vi "VendingMachine.vi"() -> ()   [LabVIEW 2019]
uses:
  Control_typedef.ctl
  Enum_states.ctl
panel:
  out "Progress":u8(slide) scale=0.0..100.0
  in  "?":bool
  in  "?":bool
  in  "?":bool
  in  "?":bool
  in  "?":bool
  in  "?":bool
  in  "Wallet":T1
  out "Juice":dbl(slide) scale=0.0..2000.0
  out "Water":dbl(slide) scale=0.0..2000.0
  out "Rum":dbl(slide) scale=0.0..2000.0
  out "Lime":dbl(slide) scale=0.0..2000.0
  out "Sugar":dbl(slide) scale=0.0..2000.0
  out "Coke":dbl(slide) scale=0.0..2000.0
  out "Whisky":dbl(slide) scale=0.0..2000.0
  in  "?":bool
  in  "?":bool
  in  "Maintainance":bool
  out "string cluster":T2
  out "Boolean":bool
  in  "ON/OFF":bool
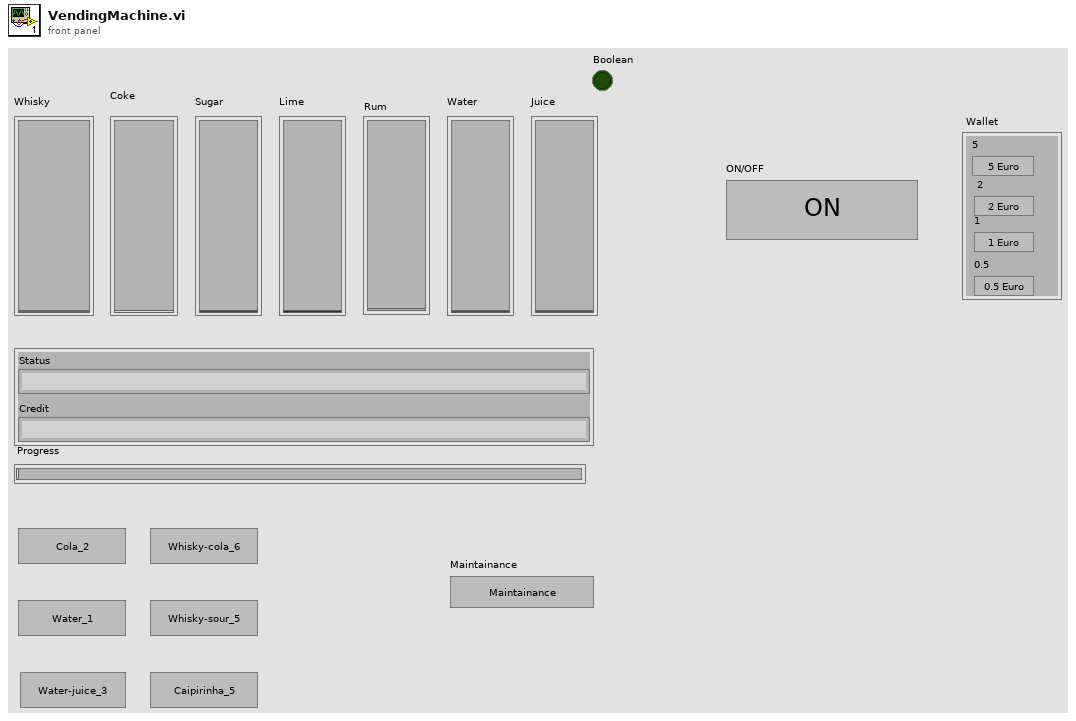
[diagram p1: front panel]
types:
  T1 = cluster{"5":bool, " 2":bool, "1":bool, "0.5":bool}
  T2 = typedef "Control_typedef.ctl" = cluster{"Status":string, "Credit":string}
  T3 = typedef "Enum_states.ctl" = enum16{"Cola-WaitMessage", "caipirinha", "whisky-sour", "whisky-cola", "water-juice", "water", "cola", "add0.5", "add1", "add2", "add5", "initialize", "OFF", "Admin mode", "Refill", "stop"}
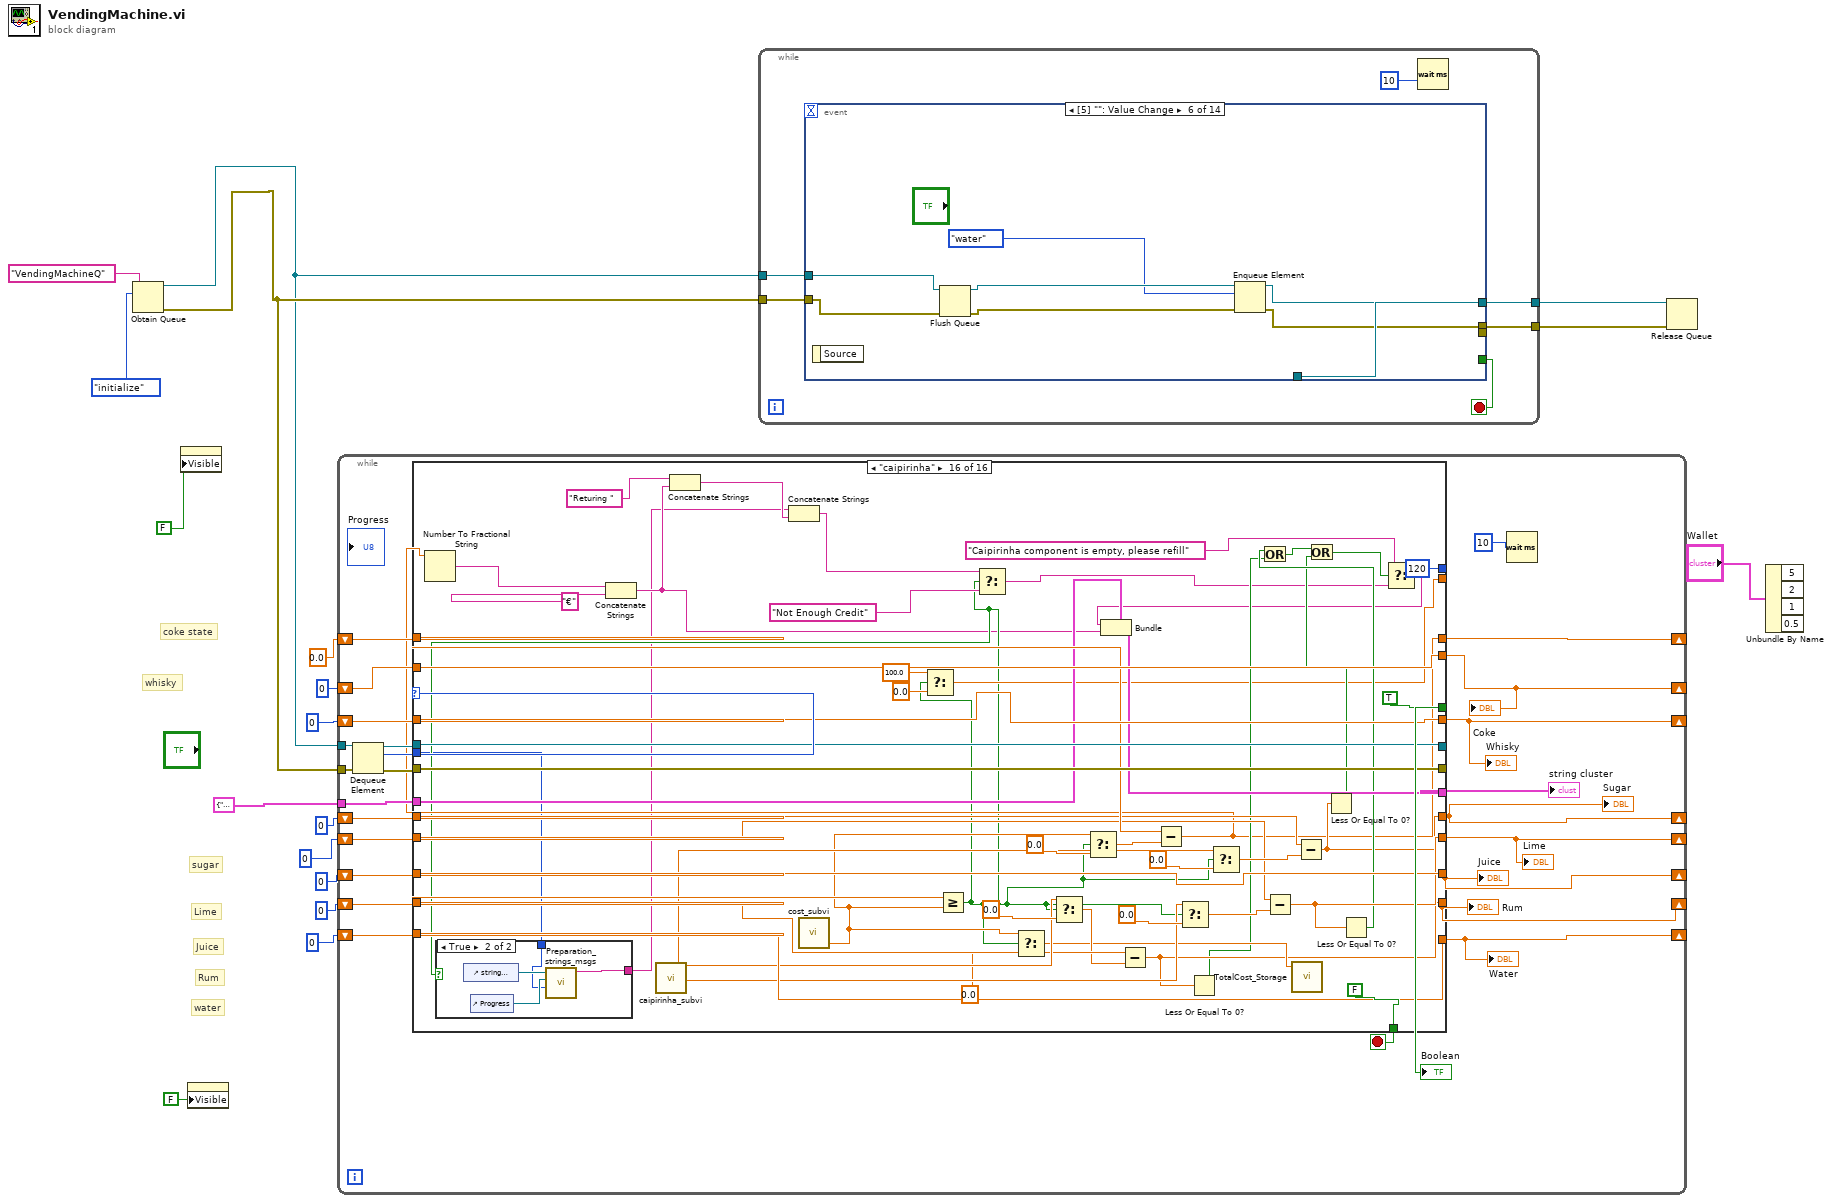
[diagram p0: block diagram]
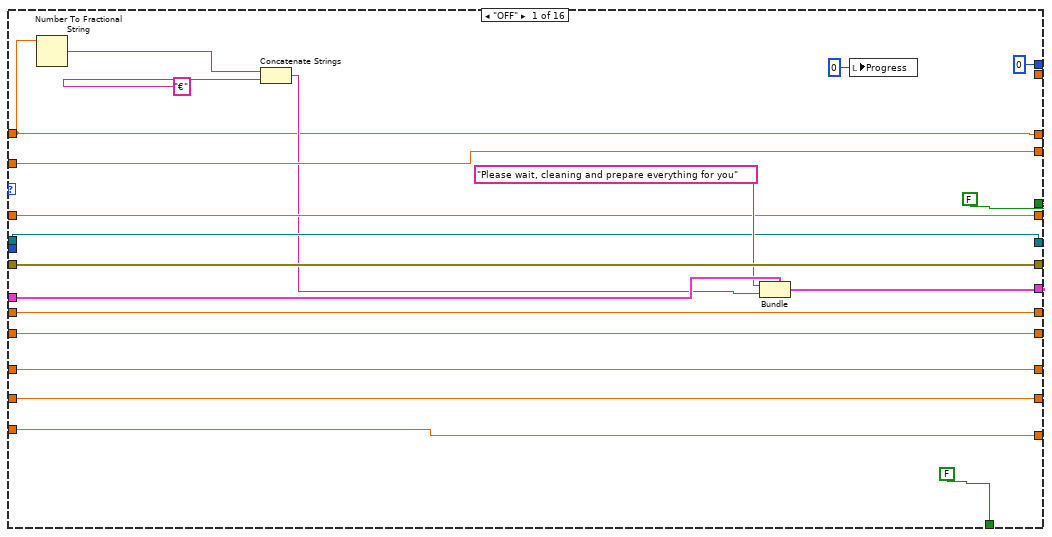
[diagram p2: hidden frame]
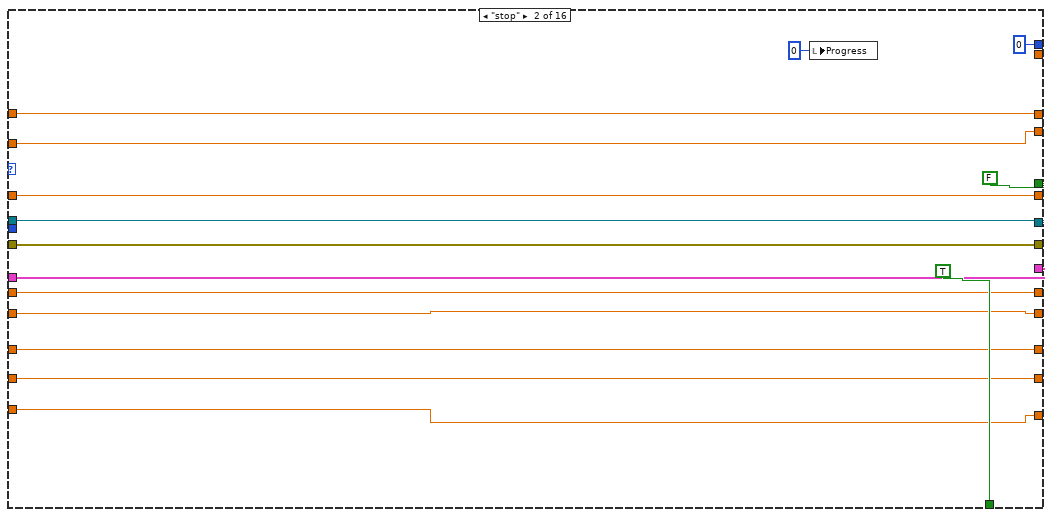
[diagram p3: hidden frame]
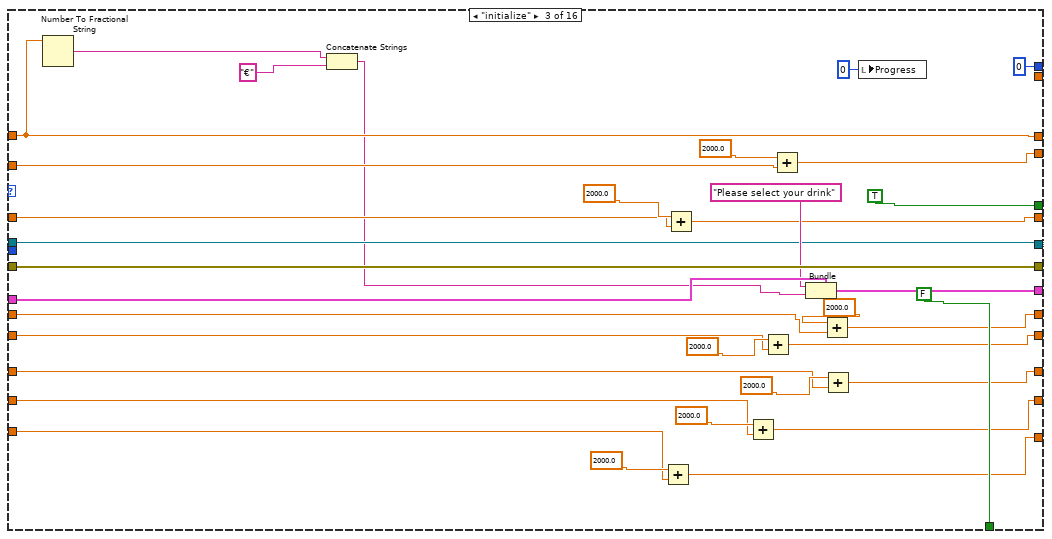
[diagram p4: hidden frame]
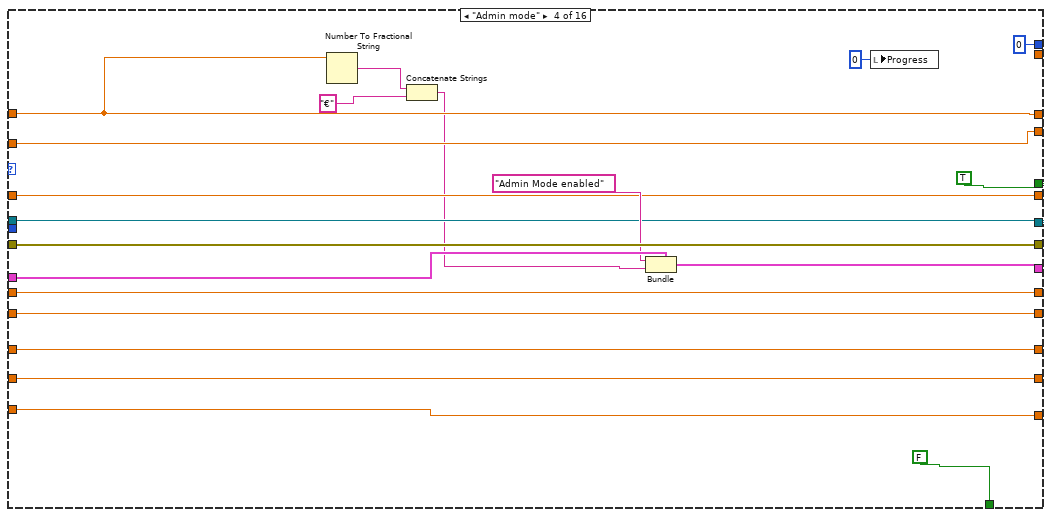
[diagram p5: hidden frame]
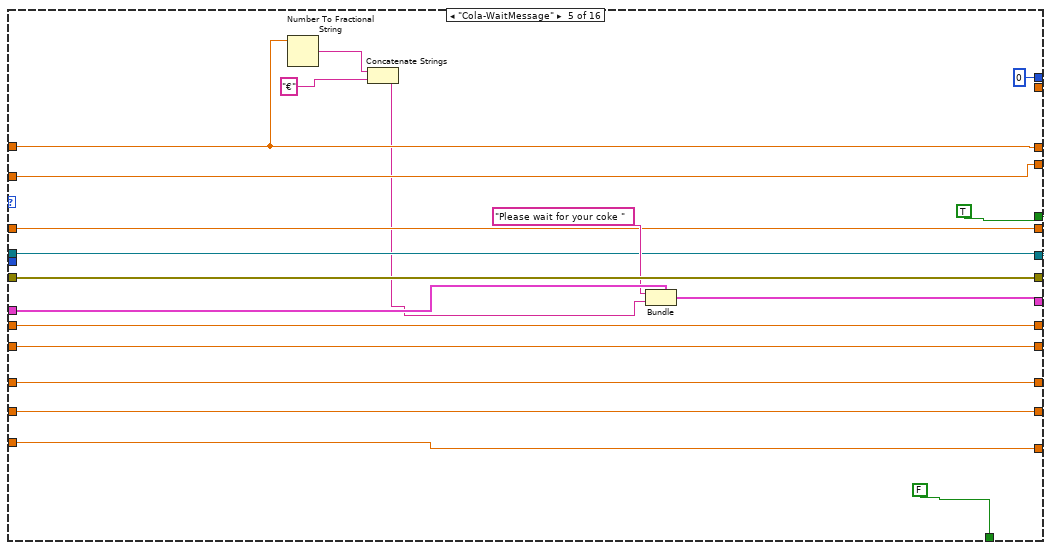
[diagram p6: hidden frame]
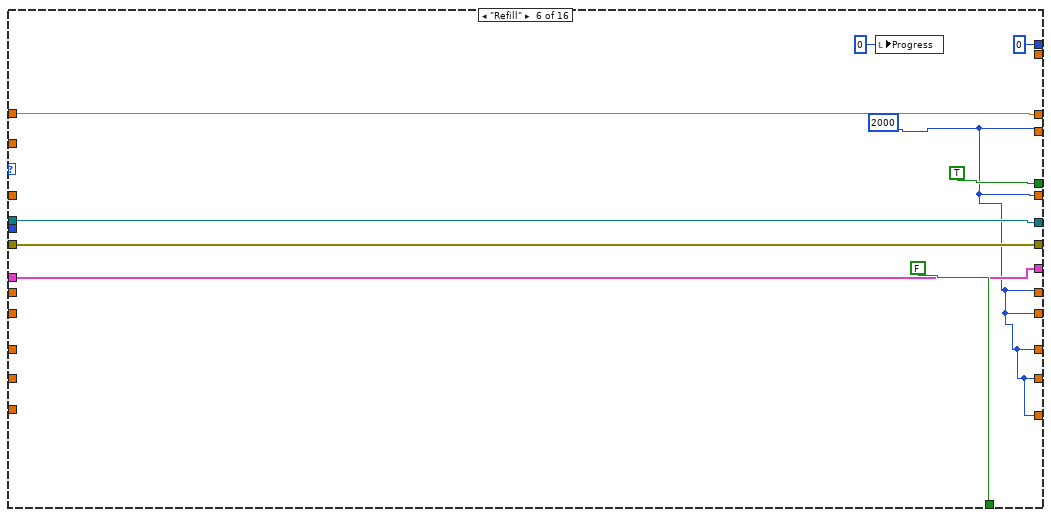
[diagram p7: hidden frame]
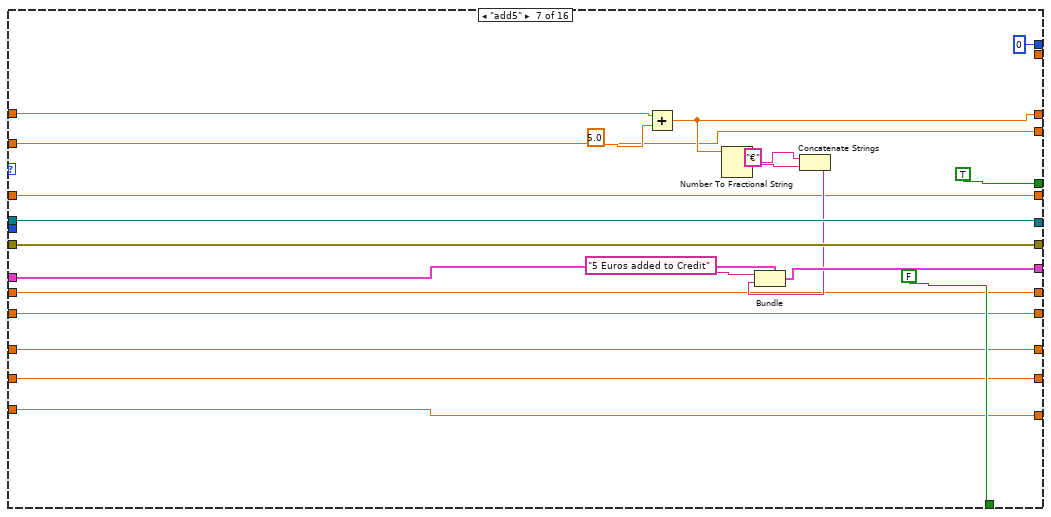
[diagram p8: hidden frame]
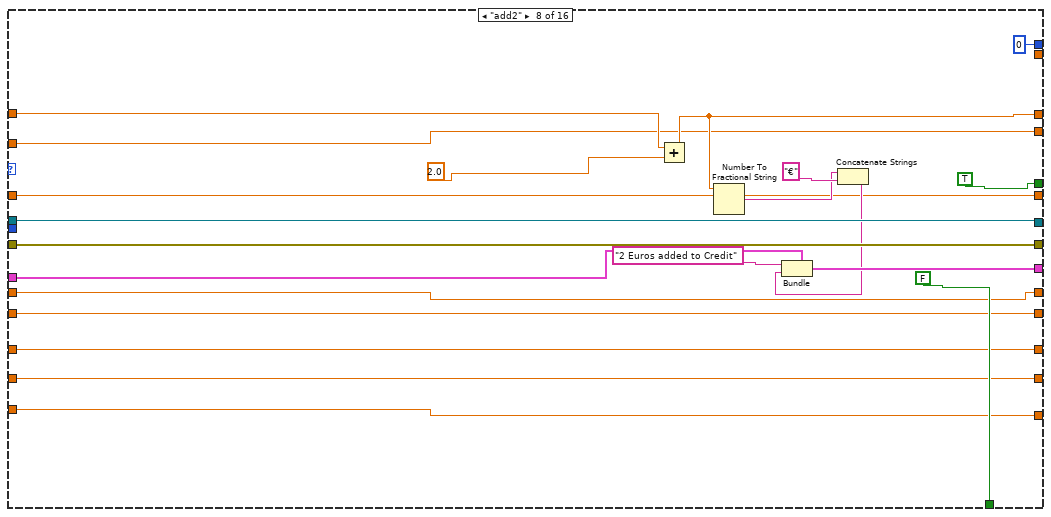
[diagram p9: hidden frame]
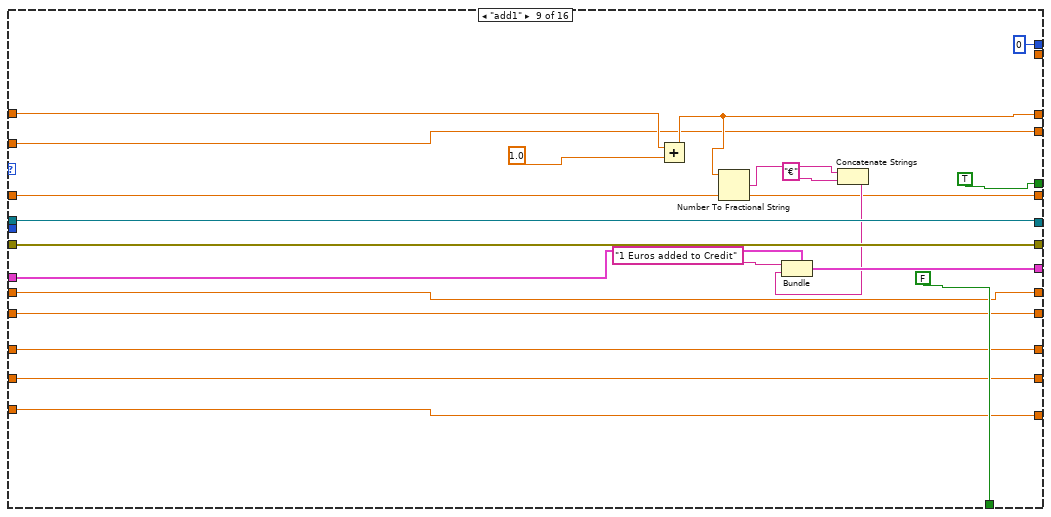
[diagram p10: hidden frame]
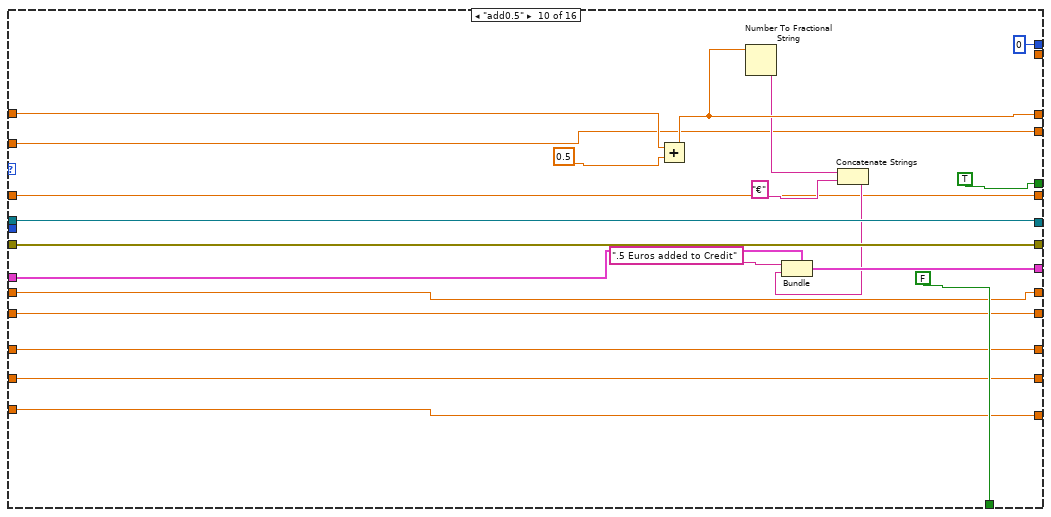
[diagram p11: hidden frame]
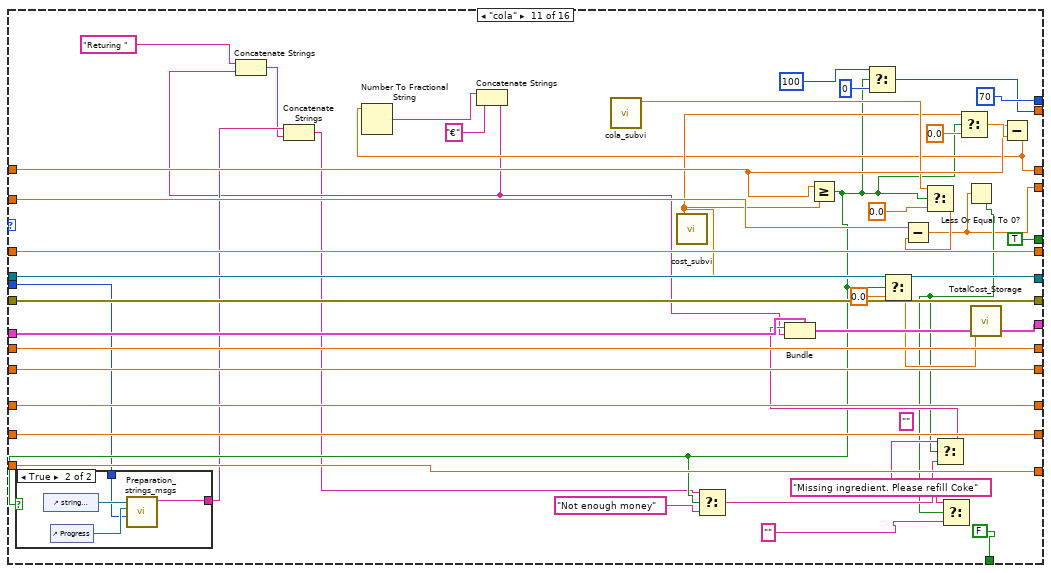
[diagram p12: hidden frame]
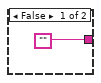
[diagram p13: hidden frame]
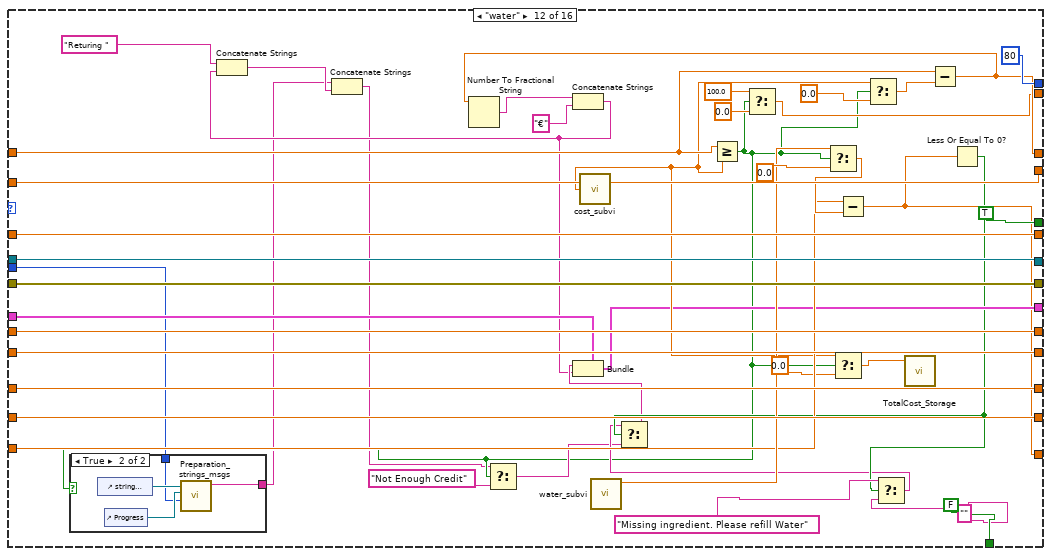
[diagram p14: hidden frame]
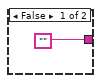
[diagram p15: hidden frame]
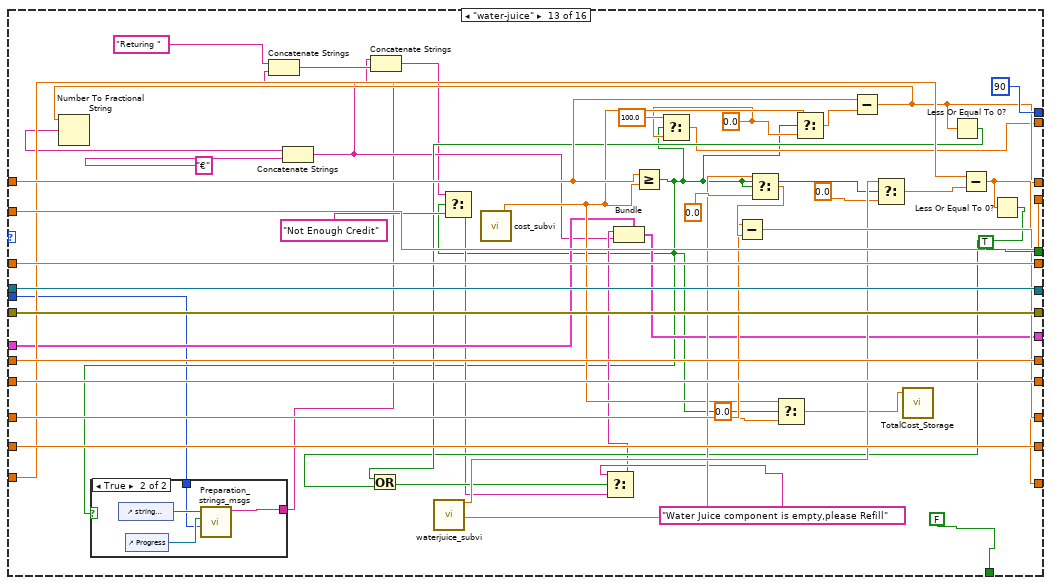
[diagram p16: hidden frame]
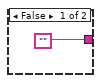
[diagram p17: hidden frame]
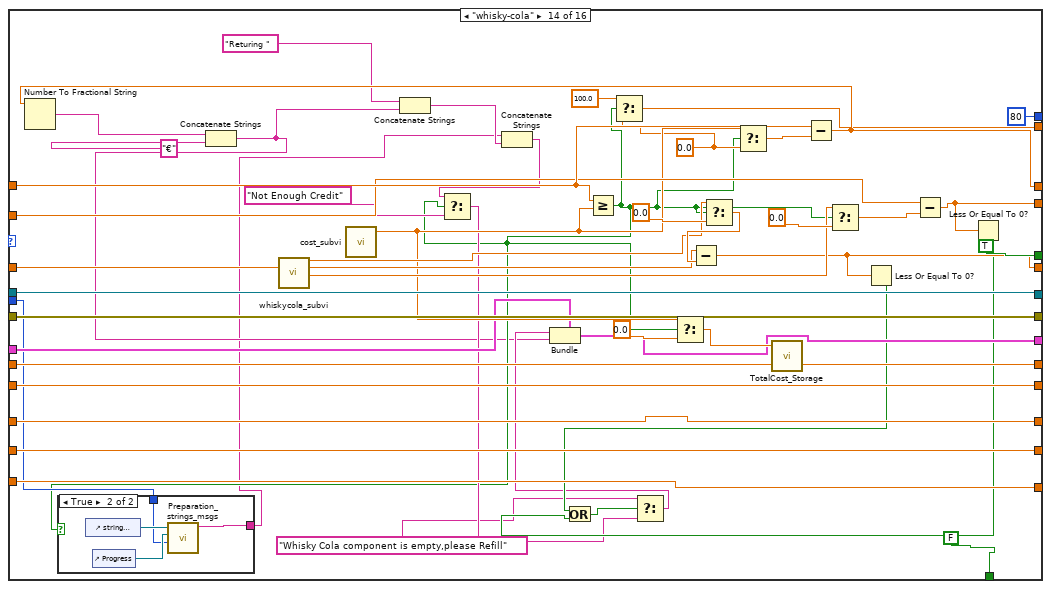
[diagram p18: hidden frame]
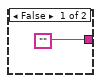
[diagram p19: hidden frame]
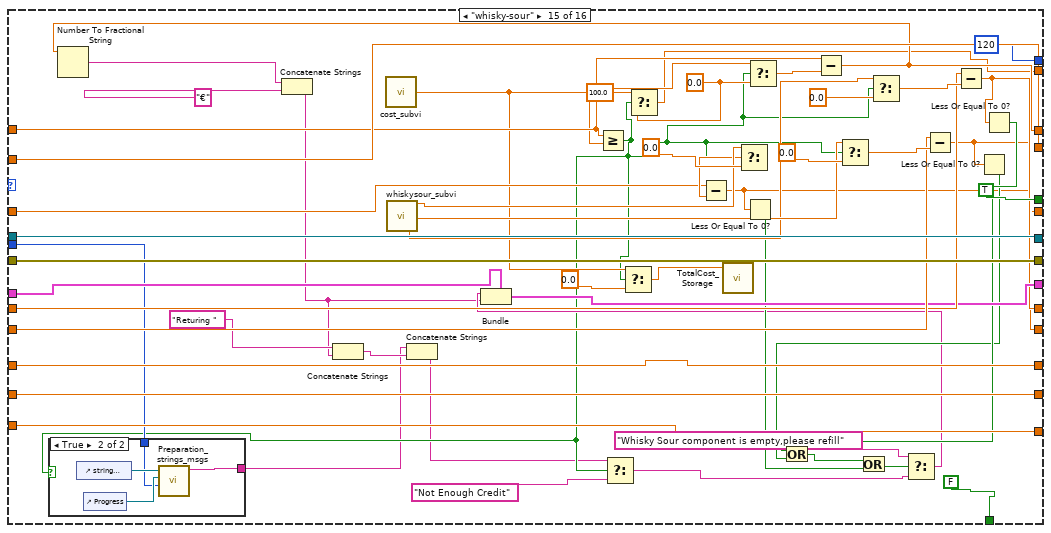
[diagram p20: hidden frame]
diagram:
  # "whisky"
  # "water"
  # "Rum"
  # "Juice"
  # "Lime"
  # "sugar"
  # "coke state"
  n1 = Obtain Queue(name (unnamed)="VendingMachineQ", element data type=Enum_states."initialize") -> (queue out=w12:refnum<queue>, error out=w13:errorcluster)  [unwired: 3 in, 1 out]
  n2 = property class="Bool"("Visible"=FALSE) -> ()  [unwired: 2 in, 2 out]
  n3 = property class="Bool"("Visible"=FALSE) -> ()  [unwired: 2 in, 2 out]
  n4 = while {
    tunnel: w12 -> [w44]
    tunnel: w13 -> [w43]
    tunnel: cluster{string, string} {"", ""} -> [w39]
    shift-right: [w35] -> _
    shift-left: 0.0 -> [w34]
    shift-right: [w32] -> _
    shift-left: 0 -> [w33]
    shift-right: [w26] -> _
    shift-left: 0 -> [w31]
    shift-right: [w27] -> _
    shift-left: 0 -> [w30]
    shift-right: [w28] -> _
    shift-left: 0 -> [w29]
    shift-right: [w24] -> _
    shift-left: 0 -> [w25]
    shift-right: [w22] -> _
    shift-left: 0 -> [w23]
    shift-right: [w20] -> _
    shift-left: 0 -> [w21]
    stop <- w37 stop-if-true
    n5 = Dequeue Element(queue=w44, error in (no error)=w43) -> (queue out=w41:refnum<queue>, element=w36:T3, error out=w40:errorcluster)  [unwired: 1 in, 1 out]
    n6 = case shown="\"caipirinha\"" w36 {
      tunnel: [FALSE FALSE TRUE TRUE TRUE TRUE TRUE TRUE TRUE TRUE TRUE TRUE TRUE TRUE TRUE TRUE] -> w42
      tunnel: w41 -> [w59 w75 w108 w128 w147 w160 w182 w203 w224 w245 w288 w337 w389 w433 w493 w554]
      tunnel: w40 -> [w64 w76 w112 w133 w152 w161 w181 w202 w223 w244 w287 w336 w388 w441 w499 w558]
      tunnel: [w64 w76 w112 w133 w152 w161 w181 w202 w223 w244 w287 w336 w388 w441 w499 w558] -> _
      tunnel: w39 -> [w63 w77 w111 w130 w149 w157 w176 w197 w218 w239 w271 w317 w365 w418 w474 w531]
      tunnel: [w62 w77 w109 w131 w150 w157 w175 w196 w217 w238 w270 w316 w364 w417 w473 w530] -> w38
      tunnel: [FALSE TRUE FALSE FALSE FALSE FALSE FALSE FALSE FALSE FALSE FALSE FALSE FALSE FALSE FALSE FALSE] -> w37
      tunnel: [w59 w75 w108 w128 w147 w160 w182 w203 w224 w245 w288 w337 w389 w433 w493 w554] -> _
      tunnel: [w54 w70 w104 w123 w142 w155 w166 w190 w208 w232 w260 w325 w383 w414 w492 w553] -> w32
      tunnel: w36 -> [_ _ _ _ _ _ _ _ _ _ w252 w300 w348 w401 w453 w510]
      tunnel: w34 -> [w46 w74 w82 w116 w135 w156 w177 w199 w220 w241 w273 w323 w377 w427 w487 w544]
      tunnel: [w46 w74 w82 w116 w135 w156 w171 w192 w213 w234 w258 w306 w353 w406 w458 w516] -> w35
      tunnel: w33 -> [w54 w70 w105 w123 w142 _ w166 w190 w208 w232 w284 w325 w383 w423 w492 w553]
      tunnel: w31 -> [w57 w73 w90 w126 w145 _ w169 w189 w211 w231 w283 w333 w385 w438 w478 w537]
      tunnel: w30 -> [w56 w72 w96 w125 w144 _ w168 w188 w210 w230 w282 w332 w376 w434 w494 w539]
      tunnel: [w55 w71 w98 w124 w143 w155 w167 w187 w209 w229 w281 w331 w384 w437 w496 w527] -> w28
      tunnel: w29 -> [w55 w71 w99 w124 w143 _ w167 w187 w209 w229 w281 w331 w384 w437 w496 w542]
      tunnel: [w56 w72 w95 w125 w144 w155 w168 w188 w210 w230 w282 w332 w375 w434 w494 w539] -> w27
      tunnel: [w57 w73 w89 w126 w145 w155 w169 w189 w211 w231 w283 w333 w385 w438 w471 w524] -> w26
      tunnel: w25 -> [w53 w69 w87 w122 w141 _ w165 w186 w207 w228 w280 w330 w382 w425 w484 w552]
      tunnel: [w53 w69 w86 w122 w141 w155 w165 w186 w207 w228 w280 w330 w382 w416 w466 w552] -> w24
      tunnel: w23 -> [w52 w68 w102 w121 w140 _ w164 w185 w206 w227 w279 w321 w370 w435 w495 w555]
      tunnel: [w52 w68 w101 w121 w140 w155 w164 w185 w206 w227 w279 w314 w363 w435 w495 w555] -> w22
      tunnel: w21 -> [w51 w67 w93 w120 w139 _ w163 w184 w205 w226 w278 w329 w381 w436 w482 w536]
      tunnel: [w51 w67 w92 w120 w139 w155 w163 w184 w205 w226 w278 w329 w381 w436 w469 w529] -> w20
      tunnel: [u32 0 ("milliseconds to wait") u32 0 ("milliseconds to wait") u32 0 ("milliseconds to wait") u32 0 ("milliseconds to wait") u32 0 ("milliseconds to wait") u32 0 ("milliseconds to wait") u32 0 ("milliseconds to wait") u32 0 ("milliseconds to wait") u32 0 ("milliseconds to wait") u32 0 ("milliseconds to wait") u32 70 ("milliseconds to wait") u32 80 ("milliseconds to wait") u32 90 ("milliseconds to wait") u32 80 ("milliseconds to wait") u32 120 ("milliseconds to wait") u32 120 ("milliseconds to wait")] -> _
      tunnel: [_ _ _ _ _ _ _ _ _ _ w255 w303 w350 w402 w454 w512] -> _
      frame "OFF" {
        n7 = Number To Fractional String(number=w46) -> (F-format string=w48:string)  [unwired: 3 in]
        n8 = Concatenate Strings(w48, "€" ("string")) -> (w47:string)
        n9 = Bundle(cluster=w63, "Please wait, cleaning and prepare everything for you", w47) -> (w62:cluster{string, string})
        n10 = local write "Progress"(u8 0 ("Progress")) -> ()
      }
      frame "stop" {
        n11 = local write "Progress"(u8 0 ("Progress")) -> ()
      }
      frame "initialize" {
        n12 = Number To Fractional String(number=w82) -> (F-format string=w83:string)  [unwired: 3 in]
        n13 = Concatenate Strings(w83, "€" ("string")) -> (w81:string)
        n14 = Add(x=2000.0, y=w102) -> (x+y=w101:dbl)
        n15 = Add(x=2000.0, y=w87) -> (x+y=w86:dbl)
        n16 = Add(x=2000.0, y=w99) -> (x+y=w98:dbl)
        n17 = Add(x=2000.0, y=w93) -> (x+y=w92:dbl)
        n18 = Add(x=2000.0, y=w105) -> (x+y=w104:dbl)
        n19 = Bundle(cluster=w111, "Please select your drink", w81) -> (w109:cluster{string, string})
        n20 = Add(x=2000.0, y=w90) -> (x+y=w89:dbl)
        n21 = Add(x=2000.0, y=w96) -> (x+y=w95:dbl)
        n22 = local write "Progress"(u8 0 ("Progress")) -> ()
      }
      frame "Admin mode" {
        n23 = Number To Fractional String(number=w116) -> (F-format string=w117:string)  [unwired: 3 in]
        n24 = Concatenate Strings(w117, "€" ("string")) -> (w115:string)
        n25 = Bundle(cluster=w130, "Admin Mode enabled", w115) -> (w131:cluster{string, string})
        n26 = local write "Progress"(u8 0 ("Progress")) -> ()
      }
      frame "Cola-WaitMessage" {
        n27 = Number To Fractional String(number=w135) -> (F-format string=w136:string)  [unwired: 3 in]
        n28 = Concatenate Strings(w136, "€" ("string")) -> (w134:string)
        n29 = Bundle(cluster=w149, "Please wait for your coke ", w134) -> (w150:cluster{string, string})
      }
      frame "Refill" {
        w155 = 2000
        n30 = local write "Progress"(u8 0 ("Progress")) -> ()
      }
      frame "add5" {
        n31 = Add(x=w177, y=5.0) -> (x+y=w171:dbl)
        n32 = Number To Fractional String(number=w171) -> (F-format string=w170:string)  [unwired: 3 in]
        n33 = Concatenate Strings(w170, "€" ("string")) -> (w172:string)
        n34 = Bundle(cluster=w176, "5 Euros added to Credit", w172) -> (w175:cluster{string, string})
      }
      frame "add2" {
        n35 = Add(x=w199, y=2.0) -> (x+y=w192:dbl)
        n36 = Number To Fractional String(number=w192) -> (F-format string=w191:string)  [unwired: 3 in]
        n37 = Concatenate Strings(w191, "€" ("string")) -> (w195:string)
        n38 = Bundle(cluster=w197, "2 Euros added to Credit", w195) -> (w196:cluster{string, string})
      }
      frame "add1" {
        n39 = Add(x=w220, y=1.0) -> (x+y=w213:dbl)
        n40 = Number To Fractional String(number=w213) -> (F-format string=w212:string)  [unwired: 3 in]
        n41 = Concatenate Strings(w212, "€" ("string")) -> (w216:string)
        n42 = Bundle(cluster=w218, "1 Euros added to Credit", w216) -> (w217:cluster{string, string})
      }
      frame "add0.5" {
        n43 = Add(x=w241, y=0.5) -> (x+y=w234:dbl)
        n44 = Number To Fractional String(number=w234) -> (F-format string=w233:string)  [unwired: 3 in]
        n45 = Concatenate Strings(w233, "€" ("string")) -> (w237:string)
        n46 = Bundle(cluster=w239, ".5 Euros added to Credit", w237) -> (w238:cluster{string, string})
      }
      frame "cola" {
        (unwired) ""
        w263 = "Missing ingredient. Please refill Coke"
        n47 = call "cola_subvi.vi"() -> ("volume"=w272:dbl)  [unwired: 9 in, 2 out]
        n48 = call "cost_subvi.vi"() -> ("Cola"=w268:dbl)  [unwired: 5 out]
        n49 = Greater Or Equal?(x=w273, y=w268) -> (x >= y?=w253:bool)
        n50 = case shown="True" w253 {
          tunnel: ["" w292] -> w251
          tunnel: w252 -> [_ w290]
          frame False {
          }
          frame True {
            n51 = control-ref of="string cluster"() -> (w293:refnum<vi>)
            n52 = control-ref of="Progress"() -> (w291:refnum<vi>)
            n53 = call "Preparation_strings_msgs.vi"("Enum"=w290, "reference"=w291, "Cluster in"=w293) -> ("Status"=w292:string)  [unwired: 8 in]
          }
        }
        n54 = Select(t=100, s=w253, f=0) -> (s? t:f=w255:i32)
        n55 = Select(t=w268, s=w253, f=0.0) -> (s? t:f=w266:dbl)
        n56 = Select(t=w272, s=w253, f=0.0) -> (s? t:f=w276:dbl)
        n57 = Subtract(x=w284, y=w276) -> (x-y=w260:dbl)
        n58 = Select(t=w268, s=w253, f=0.0) -> (s? t:f=w274:dbl)
        n59 = Less Or Equal To 0?(x=w260) -> (x <= 0?=w261:bool)
        n60 = Select(t=w263, s=w261, f="") -> ()  [unwired: 1 out]
        n61 = call "TotalCost_Storage.vi"("Numeric"=w266) -> ()  [unwired: 11 in]
        n62 = Subtract(x=w273, y=w274) -> (x-y=w258:dbl)
        n63 = Number To Fractional String(number=w258) -> (F-format string=w257:string)  [unwired: 3 in]
        n64 = Concatenate Strings(w257, "€" ("string")) -> (w249:string)
        n65 = Concatenate Strings("Returing " ("string"), w249) -> (w247:string)
        n66 = Concatenate Strings(w251, w247) -> (w246:string)
        n67 = Select(t=w246, s=w253, f="Not enough money") -> (s? t:f=w264:string)
        n68 = Select(t=w263, s=w261, f=w264) -> (s? t:f=w262:string)
        n69 = Bundle(cluster=w271, w262, w249) -> (w270:cluster{string, string})
      }
      frame "water" {
        n70 = call "cost_subvi.vi"() -> ("Water"=w320:dbl)  [unwired: 5 out]
        n71 = call "water_subvi.vi"() -> ("volume"=w322:dbl)  [unwired: 9 in, 2 out]
        n72 = Greater Or Equal?(x=w323, y=w320) -> (x >= y?=w299:bool)
        n73 = case shown="True" w299 {
          tunnel: ["" w341] -> w295
          tunnel: w300 -> [_ w339]
          frame False {
          }
          frame True {
            n74 = control-ref of="string cluster"() -> (w342:refnum<vi>)
            n75 = control-ref of="Progress"() -> (w340:refnum<vi>)
            n76 = call "Preparation_strings_msgs.vi"("Enum"=w339, "reference"=w340, "Cluster in"=w342) -> ("Status"=w341:string)  [unwired: 8 in]
          }
        }
        n77 = Select(t=100.0, s=w299, f=0.0) -> (s? t:f=w303:dbl)
        n78 = Select(t=w322, s=w299, f=0.0) -> (s? t:f=w324:dbl)
        n79 = Select(t=w320, s=w299, f=0.0) -> (s? t:f=w318:dbl)
        n80 = Subtract(x=w321, y=w324) -> (x-y=w314:dbl)
        n81 = Select(t=w320, s=w299, f=0.0) -> (s? t:f=w326:dbl)
        n82 = call "TotalCost_Storage.vi"("Numeric"=w318) -> ()  [unwired: 11 in]
        n83 = Subtract(x=w323, y=w326) -> (x-y=w306:dbl)
        n84 = Number To Fractional String(number=w306) -> (F-format string=w305:string)  [unwired: 3 in]
        n85 = Concatenate Strings(w305, "€" ("string")) -> (w297:string)
        n86 = Concatenate Strings("Returing " ("string"), w297) -> (w296:string)
        n87 = Concatenate Strings(w295, w296) -> (w294:string)
        n88 = Select(t=w294, s=w299, f="Not Enough Credit") -> (s? t:f=w309:string)
        n89 = Less Or Equal To 0?(x=w314) -> (x <= 0?=w311:bool)
        n90 = Select(t="Missing ingredient. Please refill Water" ("f"), s=w311, f="") -> (s? t:f=w310:string)
        n91 = Select(t=w310, s=w311, f=w309) -> (s? t:f=w308:string)
        n92 = Bundle(cluster=w317, w308, w297) -> (w316:cluster{string, string})
      }
      frame "water-juice" {
        w351 = 0.0 ("f")
        n93 = call "waterjuice_subvi.vi"() -> ("water quantity"=w374:dbl, "juicequantity"=w372:dbl)  [unwired: 14 in, 4 out]
        n94 = call "cost_subvi.vi"() -> ("Whater-juice"=w369:dbl)  [unwired: 5 out]
        n95 = Greater Or Equal?(x=w377, y=w369) -> (x >= y?=w349:bool)
        n96 = case shown="True" w349 {
          tunnel: ["" w393] -> w344
          tunnel: w348 -> [_ w391]
          frame False {
          }
          frame True {
            n97 = control-ref of="string cluster"() -> (w394:refnum<vi>)
            n98 = control-ref of="Progress"() -> (w392:refnum<vi>)
            n99 = call "Preparation_strings_msgs.vi"("Enum"=w391, "reference"=w392, "Cluster in"=w394) -> ("Status"=w393:string)  [unwired: 8 in]
          }
        }
        n100 = Select(t=100.0, s=w349, f=w351) -> (s? t:f=w350:dbl)
        n101 = Select(t=w372, s=w349, f=0.0) -> (s? t:f=w378:dbl)
        n102 = Subtract(x=w376, y=w378) -> (x-y=w375:dbl)
        n103 = Select(t=w369, s=w349, f=0.0) -> (s? t:f=w367:dbl)
        n104 = Select(t=w369, s=w349, f=w351) -> (s? t:f=w379:dbl)
        n105 = Subtract(x=w377, y=w379) -> (x-y=w353:dbl)
        n106 = Number To Fractional String(number=w353) -> (F-format string=w355:string)  [unwired: 3 in]
        n107 = Concatenate Strings(w355, "€" ("string")) -> (w346:string)
        n108 = Concatenate Strings("Returing " ("string"), w346) -> (w345:string)
        n109 = Concatenate Strings(w344, w345) -> (w343:string)
        n110 = Select(t=w343, s=w349, f="Not Enough Credit") -> (s? t:f=w358:string)
        n111 = Select(t=w374, s=w349, f=0.0) -> (s? t:f=w371:dbl)
        n112 = call "TotalCost_Storage.vi"("Numeric"=w367) -> ()  [unwired: 11 in]
        n113 = Less Or Equal To 0?(x=w353) -> (x <= 0?=w362:bool)
        n114 = Subtract(x=w370, y=w371) -> (x-y=w363:dbl)
        n115 = Less Or Equal To 0?(x=w363) -> (x <= 0?=w361:bool)
        n116 = Or(x=w362, y=w361) -> (x .or. y?=w360:bool)
        n117 = Select(t="Water Juice component is empty,please Refill" ("f"), s=w360, f=w358) -> (s? t:f=w357:string)
        n118 = Bundle(cluster=w365, w357, w346) -> (w364:cluster{string, string})
      }
      frame "whisky-cola" {
        w403 = 0.0 ("f")
        n119 = call "whiskycola_subvi.vi"() -> ("whisk quantity"=w426:dbl, "cola quantity"=w424:dbl)  [unwired: 14 in, 4 out]
        n120 = call "cost_subvi.vi"() -> ("Whisky-cola"=w422:dbl)  [unwired: 5 out]
        n121 = Greater Or Equal?(x=w427, y=w422) -> (x >= y?=w400:bool)
        n122 = case shown="True" w400 {
          tunnel: ["" w445] -> w396
          tunnel: w401 -> [_ w443]
          frame False {
          }
          frame True {
            n123 = control-ref of="string cluster"() -> (w446:refnum<vi>)
            n124 = control-ref of="Progress"() -> (w444:refnum<vi>)
            n125 = call "Preparation_strings_msgs.vi"("Enum"=w443, "reference"=w444, "Cluster in"=w446) -> ("Status"=w445:string)  [unwired: 8 in]
          }
        }
        n126 = Select(t=100.0, s=w400, f=w403) -> (s? t:f=w402:dbl)
        n127 = Select(t=w422, s=w400, f=0.0) -> (s? t:f=w420:dbl)
        n128 = Select(t=w426, s=w400, f=0.0) -> (s? t:f=w430:dbl)
        n129 = Subtract(x=w425, y=w430) -> (x-y=w416:dbl)
        n130 = Select(t=w422, s=w400, f=w403) -> (s? t:f=w431:dbl)
        n131 = call "TotalCost_Storage.vi"("Numeric"=w420) -> ()  [unwired: 11 in]
        n132 = Subtract(x=w427, y=w431) -> (x-y=w406:dbl)
        n133 = Number To Fractional String(number=w406) -> (F-format string=w405:string)  [unwired: 3 in]
        n134 = Concatenate Strings(w405, "€" ("string")) -> (w398:string)
        n135 = Concatenate Strings("Returing " ("string"), w398) -> (w397:string)
        n136 = Concatenate Strings(w396, w397) -> (w395:string)
        n137 = Select(t=w395, s=w400, f="Not Enough Credit") -> (s? t:f=w411:string)
        n138 = Select(t=w424, s=w400, f=0.0) -> (s? t:f=w428:dbl)
        n139 = Less Or Equal To 0?(x=w416) -> (x <= 0?=w415:bool)
        n140 = Subtract(x=w423, y=w428) -> (x-y=w414:dbl)
        n141 = Less Or Equal To 0?(x=w414) -> (x <= 0?=w413:bool)
        n142 = Or(x=w415, y=w413) -> (x .or. y?=w412:bool)
        n143 = Select(t="Whisky Cola component is empty,please Refill" ("f"), s=w412, f=w411) -> (s? t:f=w409:string)
        n144 = Bundle(cluster=w418, w409, w398) -> (w417:cluster{string, string})
      }
      frame "whisky-sour" {
        w456 = 0.0 ("f")
        n145 = call "cost_subvi.vi"() -> ("Whisky-sour"=w477:dbl)  [unwired: 5 out]
        n146 = call "whiskysour_subvi.vi"() -> ("sugar qntity"=w479:dbl, "whisky quantity"=w486:dbl, "lime quantity"=w483:dbl)  [unwired: 11 in, 6 out]
        n147 = Greater Or Equal?(x=w487, y=w477) -> (x >= y?=w452:bool)
        n148 = case shown="True" w452 {
          tunnel: ["" w503] -> w448
          tunnel: w453 -> [_ w501]
          frame False {
          }
          frame True {
            n149 = control-ref of="string cluster"() -> (w504:refnum<vi>)
            n150 = control-ref of="Progress"() -> (w502:refnum<vi>)
            n151 = call "Preparation_strings_msgs.vi"("Enum"=w501, "reference"=w502, "Cluster in"=w504) -> ("Status"=w503:string)  [unwired: 8 in]
          }
        }
        n152 = Select(t=w477, s=w452, f=0.0) -> (s? t:f=w475:dbl)
        n153 = Select(t=100.0, s=w452, f=w456) -> (s? t:f=w454:dbl)
        n154 = call "TotalCost_Storage.vi"("Numeric"=w475) -> ()  [unwired: 11 in]
        n155 = Select(t=w486, s=w452, f=0.0) -> (s? t:f=w485:dbl)
        n156 = Subtract(x=w484, y=w485) -> (x-y=w466:dbl)
        n157 = Less Or Equal To 0?(x=w466) -> (x <= 0?=w465:bool)
        n158 = Select(t=w477, s=w452, f=w456) -> (s? t:f=w490:dbl)
        n159 = Subtract(x=w487, y=w490) -> (x-y=w458:dbl)
        n160 = Number To Fractional String(number=w458) -> (F-format string=w457:string)  [unwired: 3 in]
        n161 = Concatenate Strings(w457, "€" ("string")) -> (w450:string)
        n162 = Concatenate Strings("Returing " ("string"), w450) -> (w449:string)
        n163 = Concatenate Strings(w448, w449) -> (w447:string)
        n164 = Select(t=w447, s=w452, f="Not Enough Credit") -> (s? t:f=w463:string)
        n165 = Select(t=w483, s=w452, f=0.0) -> (s? t:f=w488:dbl)
        n166 = Select(t=w479, s=w452, f=0.0) -> (s? t:f=w480:dbl)
        n167 = Subtract(x=w482, y=w488) -> (x-y=w469:dbl)
        n168 = Subtract(x=w478, y=w480) -> (x-y=w471:dbl)
        n169 = Less Or Equal To 0?(x=w469) -> (x <= 0?=w468:bool)
        n170 = Less Or Equal To 0?(x=w471) -> (x <= 0?=w470:bool)
        n171 = Or(x=w470, y=w468) -> (x .or. y?=w467:bool)
        n172 = Or(x=w467, y=w465) -> (x .or. y?=w464:bool)
        n173 = Select(t="Whisky Sour component is empty,please refill", s=w464, f=w463) -> (s? t:f=w461:string)
        n174 = Bundle(cluster=w474, w461, w450) -> (w473:cluster{string, string})
      }
      frame "caipirinha" {
        n175 = call "caipirinha_subvi.vi"() -> ("sugar qntity"=w538:dbl, "rum quantity"=w543:dbl, "lime quantity"=w540:dbl)  [unwired: 11 in, 6 out]
        n176 = call "cost_subvi.vi"() -> ("capirinha"=w535:dbl)  [unwired: 5 out]
        n177 = Greater Or Equal?(x=w544, y=w535) -> (x >= y?=w511:bool)
        n178 = case shown="True" w511 {
          tunnel: ["" w562] -> w506
          tunnel: w510 -> [_ w560]
          frame False {
          }
          frame True {
            n179 = control-ref of="string cluster"() -> (w563:refnum<vi>)
            n180 = control-ref of="Progress"() -> (w561:refnum<vi>)
            n181 = call "Preparation_strings_msgs.vi"("Enum"=w560, "reference"=w561, "Cluster in"=w563) -> ("Status"=w562:string)  [unwired: 8 in]
          }
        }
        n182 = Select(t=100.0, s=w511, f=0.0) -> (s? t:f=w512:dbl)
        n183 = Select(t=w535, s=w511, f=0.0) -> (s? t:f=w533:dbl)
        n184 = Select(t=w543, s=w511, f=0.0) -> (s? t:f=w541:dbl)
        n185 = Select(t=w535, s=w511, f=0.0) -> (s? t:f=w549:dbl)
        n186 = Subtract(x=w542, y=w541) -> (x-y=w527:dbl)
        n187 = Subtract(x=w544, y=w549) -> (x-y=w516:dbl)
        n188 = Number To Fractional String(number=w516) -> (F-format string=w515:string)  [unwired: 3 in]
        n189 = Concatenate Strings(w515, "€" ("string")) -> (w508:string)
        n190 = Concatenate Strings("Returing " ("string"), w508) -> (w507:string)
        n191 = Concatenate Strings(w506, w507) -> (w505:string)
        n192 = Select(t=w505, s=w511, f="Not Enough Credit") -> (s? t:f=w521:string)
        n193 = Select(t=w540, s=w511, f=0.0) -> (s? t:f=w547:dbl)
        n194 = Less Or Equal To 0?(x=w527) -> (x <= 0?=w526:bool)
        n195 = Select(t=w538, s=w511, f=0.0) -> (s? t:f=w545:dbl)
        n196 = Subtract(x=w536, y=w547) -> (x-y=w529:dbl)
        n197 = call "TotalCost_Storage.vi"("Numeric"=w533) -> ()  [unwired: 11 in]
        n198 = Subtract(x=w537, y=w545) -> (x-y=w524:dbl)
        n199 = Less Or Equal To 0?(x=w524) -> (x <= 0?=w523:bool)
        n200 = Less Or Equal To 0?(x=w529) -> (x <= 0?=w528:bool)
        n201 = Or(x=w528, y=w526) -> (x .or. y?=w525:bool)
        n202 = Or(x=w525, y=w523) -> (x .or. y?=w522:bool)
        n203 = Select(t="Caipirinha component is empty, please refill", s=w522, f=w521) -> (s? t:f=w519:string)
        n204 = Bundle(cluster=w531, w519, w508) -> (w530:cluster{string, string})
      }
    }
    "Boolean" <- w42
    "string cluster" <- w38
    "Coke" <- w32
    "Sugar" <- w26
    "Lime" <- w20
    "Rum" <- w28
    "Water" <- w22
    "Juice" <- w27
    "Whisky" <- w24
    n205 = Wait (ms)(milliseconds to wait=u32 10) -> ()  [unwired: 1 out]
  }
  n206 = while {
    tunnel: w12 -> [w569]
    tunnel: w13 -> [w568]
    tunnel: [w567] -> w16
    tunnel: [w566] -> w15
    stop <- w565 stop-if-true
    n207 = event shown="[5] \"\": Value Change" {
      selector: _ -> [_ _ _ _ _ _ _ _ _ _ _ _ _ _]
      dyn-events: _ -> [_ _ _ _ _ _ _ _ _ _ _ _ _ _]
      timeout: _ -> [_ _ _ _ _ _ _ _ _ _ _ _ _ _]
      tunnel: w569 -> [w576 w584 w592 w605 w609 w618 w628 w636 w645 w652 w661 w667 w674 w679]
      tunnel: w568 -> [w575 w583 w591 w604 w608 w617 w627 w635 w644 w651 w660 w666 w673 w678]
      tunnel: [w572 _ _ _ w611 _ _ _ w643 w650 w659 w665 w671 _] -> w567
      tunnel: [w571 w581 w589 w601 w610 w619 w625 w633 w642 w649 w658 w664 _ w680] -> w566
      tunnel: [_ FALSE FALSE FALSE _ _ FALSE FALSE TRUE FALSE FALSE _ _ _] -> w565
      tunnel: [_ _ _ _ _ _ _ _ _ _ _ _ w672 _] -> _
      tunnel: [_ w582 w590 w602 _ w620 w626 w634 _ _ _ _ _ w681] -> _
      event "ON/OFF": Value Change {
        n208 = event-data() -> ()  [unwired: 1 in, 1 out]
        n209 = Flush Queue(queue=w576, error in (no error)=w575) -> (queue out=w574:refnum<queue>, error out=w573:errorcluster)  [unwired: 1 out]
        n210 = Select(t=Enum_states."initialize", s="ON/OFF", f=Enum_states."OFF") -> (s? t:f=w570:T3)
        n211 = Enqueue Element(queue=w574, element=w570, error in (no error)=w573) -> (queue out=w572:refnum<queue>, error out=w571:errorcluster)  [unwired: 1 in, 1 out]
      }
      event Value Change {
        n212 = event-data() -> ()  [unwired: 1 in, 1 out]
        n213 = Flush Queue(queue=w584, error in (no error)=w583) -> (queue out=w587:refnum<queue>, error out=w586:errorcluster)  [unwired: 1 out]
        n214 = Enqueue Element(queue=w587, element=Enum_states."whisky-sour", error in (no error)=w586) -> (queue out=w582:refnum<queue>, error out=w581:errorcluster)  [unwired: 1 in, 1 out]
      }
      event Value Change {
        # "s"
        n215 = event-data() -> ()  [unwired: 1 in, 1 out]
        n216 = Flush Queue(queue=w592, error in (no error)=w591) -> (queue out=w595:refnum<queue>, error out=w594:errorcluster)  [unwired: 1 out]
        n217 = Enqueue Element(queue=w595, element=Enum_states."caipirinha", error in (no error)=w594) -> (queue out=w590:refnum<queue>, error out=w589:errorcluster)  [unwired: 1 in, 1 out]
      }
      event Value Change {
        n218 = event-data() -> ()  [unwired: 1 in, 1 out]
        n219 = Flush Queue(queue=w605, error in (no error)=w604) -> (queue out=w600:refnum<queue>, error out=w606:errorcluster)  [unwired: 1 out]
        n220 = Select(t=Enum_states."Cola-WaitMessage", s=FALSE, f=Enum_states."cola") -> (s? t:f=w599:T3)
        n221 = Enqueue Element(queue=w600, element=w599, error in (no error)=w606) -> (queue out=w602:refnum<queue>, error out=w601:errorcluster)  [unwired: 1 in, 1 out]
      }
      event "Maintainance": Value Change {
        n222 = event-data() -> ()  [unwired: 1 in, 1 out]
        n223 = Flush Queue(queue=w609, error in (no error)=w608) -> (queue out=w614:refnum<queue>, error out=w613:errorcluster)  [unwired: 1 out]
        n224 = Select(t=Enum_states."Admin mode", s="Maintainance", f=Enum_states."initialize") -> (s? t:f=w612:T3)
        n225 = Enqueue Element(queue=w614, element=w612, error in (no error)=w613) -> (queue out=w611:refnum<queue>, error out=w610:errorcluster)  [unwired: 1 in, 1 out]
        n226 = property class="Bool"("Visible"="Maintainance") -> ()  [unwired: 2 in, 2 out]
        n227 = property class="Bool"("Visible"="Maintainance") -> ()  [unwired: 2 in, 2 out]
      }
      event Value Change {
        n228 = event-data() -> ()  [unwired: 1 in, 1 out]
        n229 = Flush Queue(queue=w618, error in (no error)=w617) -> (queue out=w623:refnum<queue>, error out=w622:errorcluster)  [unwired: 1 out]
        n230 = Enqueue Element(queue=w623, element=Enum_states."water", error in (no error)=w622) -> (queue out=w620:refnum<queue>, error out=w619:errorcluster)  [unwired: 1 in, 1 out]
      }
      event Value Change {
        n231 = event-data() -> ()  [unwired: 1 in, 1 out]
        n232 = Flush Queue(queue=w628, error in (no error)=w627) -> (queue out=w631:refnum<queue>, error out=w630:errorcluster)  [unwired: 1 out]
        n233 = Enqueue Element(queue=w631, element=Enum_states."water-juice", error in (no error)=w630) -> (queue out=w626:refnum<queue>, error out=w625:errorcluster)  [unwired: 1 in, 1 out]
      }
      event Value Change {
        n234 = event-data() -> ()  [unwired: 1 in, 1 out]
        n235 = Flush Queue(queue=w636, error in (no error)=w635) -> (queue out=w639:refnum<queue>, error out=w638:errorcluster)  [unwired: 1 out]
        n236 = Enqueue Element(queue=w639, element=Enum_states."whisky-cola", error in (no error)=w638) -> (queue out=w634:refnum<queue>, error out=w633:errorcluster)  [unwired: 1 in, 1 out]
      }
      event Value Change {
        n237 = event-data() -> ()  [unwired: 1 in, 1 out]
        n238 = Flush Queue(queue=w645, error in (no error)=w644) -> (queue out=w647:refnum<queue>, error out=w646:errorcluster)  [unwired: 1 out]
        n239 = Enqueue Element(queue=w647, element=Enum_states."stop", error in (no error)=w646) -> (queue out=w643:refnum<queue>, error out=w642:errorcluster)  [unwired: 1 in, 1 out]
      }
      event Value Change {
        n240 = event-data() -> ()  [unwired: 1 in, 1 out]
        n241 = Flush Queue(queue=w652, error in (no error)=w651) -> (queue out=w655:refnum<queue>, error out=w654:errorcluster)  [unwired: 1 out]
        n242 = Enqueue Element(queue=w655, element=Enum_states."Refill", error in (no error)=w654) -> (queue out=w650:refnum<queue>, error out=w649:errorcluster)  [unwired: 1 in, 1 out]
      }
      event "Wallet.5": Value Change {
        n243 = event-data() -> ()  [unwired: 1 in, 1 out]
        n244 = Flush Queue(queue=w661, error in (no error)=w660) -> (queue out=w663:refnum<queue>, error out=w662:errorcluster)  [unwired: 1 out]
        n245 = Enqueue Element(queue=w663, element=Enum_states."add5", error in (no error)=w662) -> (queue out=w659:refnum<queue>, error out=w658:errorcluster)  [unwired: 1 in, 1 out]
      }
      event "Wallet.2": Value Change {
        n246 = event-data() -> ()  [unwired: 1 in, 1 out]
        n247 = Flush Queue(queue=w667, error in (no error)=w666) -> (queue out=w670:refnum<queue>, error out=w669:errorcluster)  [unwired: 1 out]
        n248 = Enqueue Element(queue=w670, element=Enum_states."add2", error in (no error)=w669) -> (queue out=w665:refnum<queue>, error out=w664:errorcluster)  [unwired: 1 in, 1 out]
      }
      event "Wallet.1": Value Change {
        n249 = event-data() -> ()  [unwired: 1 in, 1 out]
        n250 = Flush Queue(queue=w674, error in (no error)=w673) -> (queue out=w677:refnum<queue>, error out=w676:errorcluster)  [unwired: 1 out]
        n251 = Enqueue Element(queue=w677, element=Enum_states."add1", error in (no error)=w676) -> (queue out=w671:refnum<queue>, error out=w672:errorcluster)  [unwired: 1 in, 1 out]
      }
      event "Wallet.0.5": Value Change {
        n252 = event-data() -> ()  [unwired: 1 in, 1 out]
        n253 = Flush Queue(queue=w679, error in (no error)=w678) -> (queue out=w684:refnum<queue>, error out=w683:errorcluster)  [unwired: 1 out]
        n254 = Enqueue Element(queue=w684, element=Enum_states."add0.5", error in (no error)=w683) -> (queue out=w681:refnum<queue>, error out=w680:errorcluster)  [unwired: 1 in, 1 out]
      }
    }
    n255 = Wait (ms)(milliseconds to wait=u32 10) -> ()  [unwired: 1 out]
  }
  n256 = Release Queue(queue=w16, error in (no error)=w15) -> ()  [unwired: 1 in, 3 out]
  n257 = Unbundle By Name("Wallet") -> ()  [unwired: 4 out]
